vi "Build_Asylum_WriteGroup.vi"(8 "error in (no error)":errorcluster, 10 "wave":string, 11 "groupName":string) -> (0 "error out":errorcluster, 3 "Command":string)   [LabVIEW 2019]
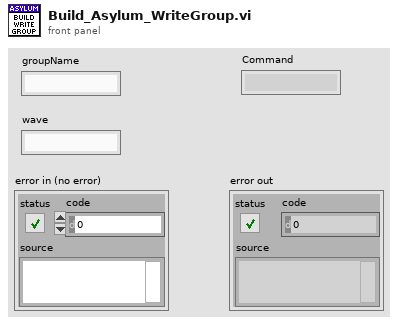
[diagram p1: front panel]
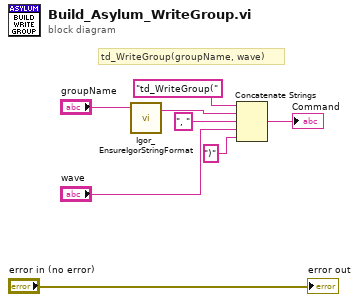
[diagram p0: block diagram]
diagram:
  # "td_WriteGroup(groupName, wave)"
  n1 = call <userlib>:"Igor_EnsureIgorStringFormat.vi"("Value"="groupName") -> ("Value"=w6:string)  [unwired: 2 in]
  n2 = Concatenate Strings("td_WriteGroup(" ("string"), w6, ", " ("string"), "wave", ")" ("string")) -> (→"Command":string)
  "error out" <- "error in (no error)"
